vi "Set3Points.vi"(0 "Counter":i32, 5 "axis id":string[](array[string]), 7 "System number":i32, 9 "stop":bool, 11 "Z Axis Step  Size":dbl, 12 "Error In":errorcluster) -> (3 "Relative Position":dbl[](array[numeric]), 6 "3Points2DArray":dbl[][](array[numeric]), 15 "Error Out":errorcluster)   [LabVIEW 2019]
uses:
  <vilib>/Analysis/Matrix/Datatypes/RealMatrix.ctl
  <vilib>/Analysis/Matrix/Numeric/Conversions/Matrix To Array - RM.vi
  <vilib>/Analysis/Matrix/NI_Matrix.lvlib
panel:
  in  "3Points":T1
  in  "zRandom":T1
  out "Iteration":i32
  out "MaxRandomNum":dbl
  out "zrandArray":dbl[][](array[numeric])
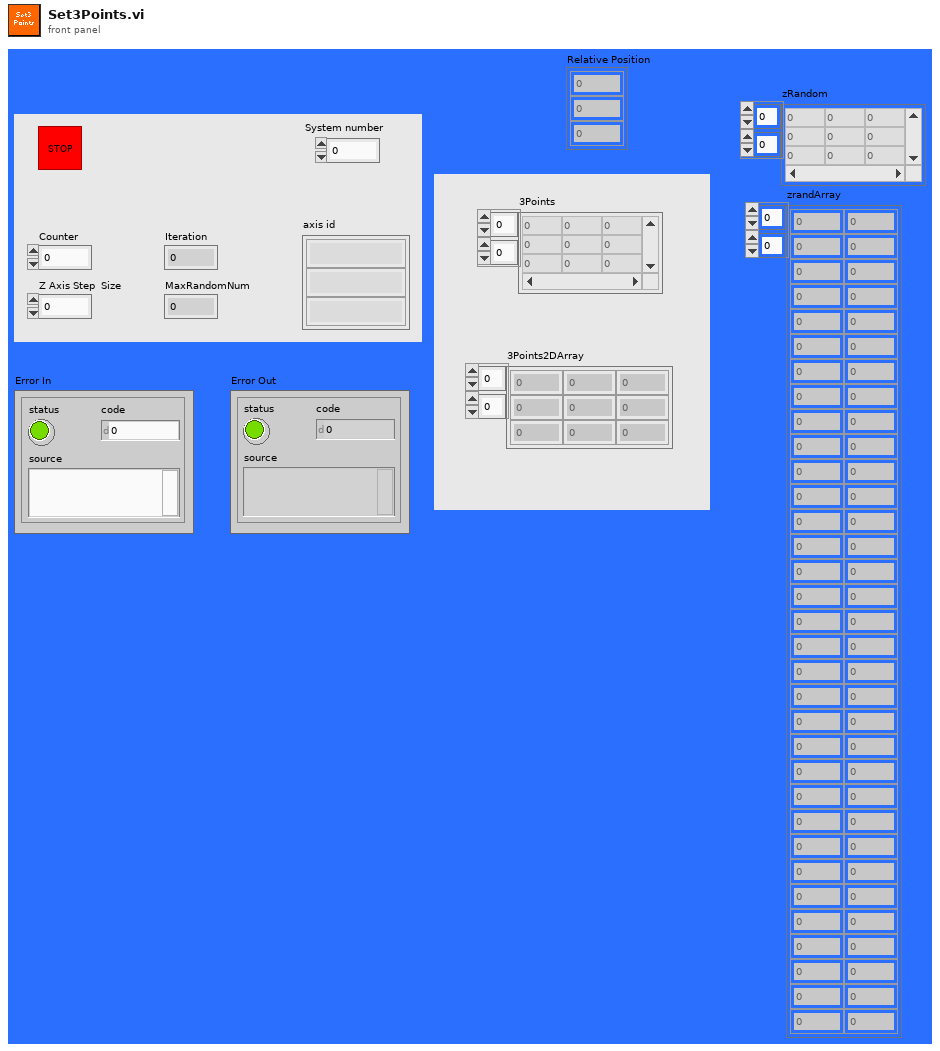
[diagram p1: front panel]
types:
  T1 = typedef "NI_Matrix.lvlib/RealMatrix.ctl" = dbl[][]
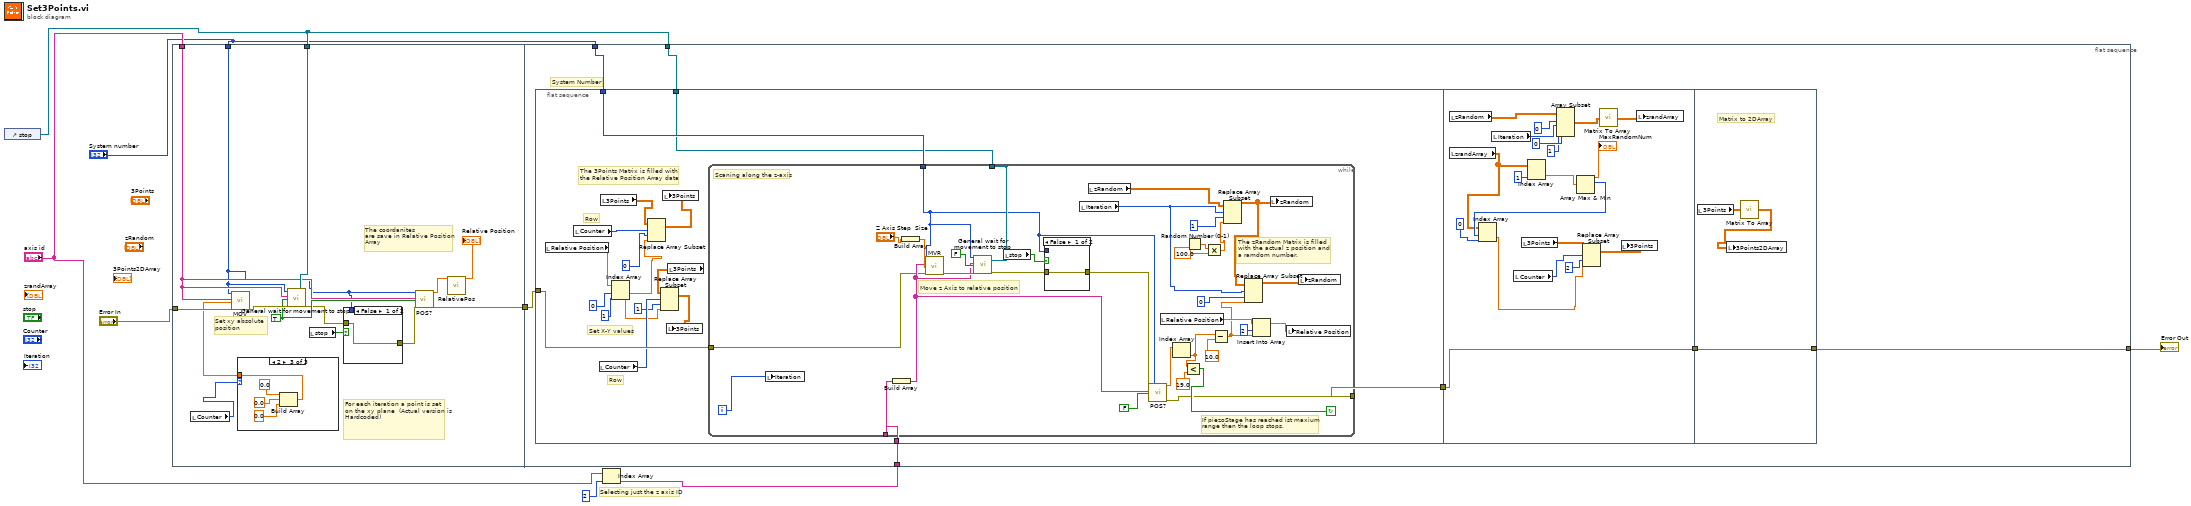
[diagram p0: block diagram]
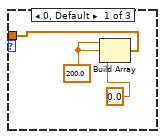
[diagram p2: hidden frame]
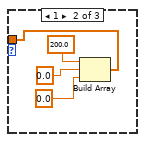
[diagram p3: hidden frame]
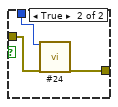
[diagram p4: hidden frame]
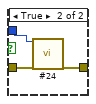
[diagram p5: hidden frame]
diagram:
  # "Selecting just the z axis ID"
  n1 = control-ref of="stop"() -> (w2:refnum<vi>)
  n2 = flat-sequence {
    tunnel: "Error In" -> [w22]
    tunnel: w2 -> [w20]
    tunnel: "axis id" -> [w18]
    tunnel: "System number" -> [w12]
    tunnel: [w19] -> w8
    tunnel: w8 -> [w44]
    tunnel: "System number" -> [w43]
    tunnel: w2 -> [w42]
    tunnel: w4 -> [w41]
    tunnel: [w39] -> w3
    frame #0 {
      w17 = TRUE ("All axes?")
      # "The coordanites\nare save in Relative Position \nArray"
      # "For each iteration a point is set\non the xy plane  (Actual version is Hardcoded)"
      # "Set xy absolute\nposition"
      n3 = local read "Counter"() -> (w9:i32)
      n4 = case shown="2" w9 {
        tunnel: [w23 w26 w30] -> w10
        frame 0, Default {
          w25 = 200.0 ("element")
          n5 = Build Array(w25, w25, 0.0 ("element")) -> (w23:dbl[])
        }
        frame 1 {
          n6 = Build Array(200.0, 0.0, 0.0) -> (w26:dbl[])
        }
        frame 2 {
          n7 = Build Array(0.0, 0.0, 0.0) -> (w30:dbl[])
        }
      }
      n8 = call "MOV.vi"("System no."=w12, "Axes to move"=w18, "Position values"=w10, "error in"=w22) -> ("error out"=w21:errorcluster)  [unwired: 15 in]
      n9 = call "General wait for movement to stop.vi"("System no."=w12, "Axes to wait for"=w18, "All axes?"=w17, "error in"=w21, "Stop refnum"=w20) -> ("error out"=w13:errorcluster)  [unwired: 13 in, 1 out]
      n10 = local read "stop"() -> (w14:bool)
      n11 = case shown="False" w14 {
        tunnel: w13 -> [w34 w37]
        tunnel: w12 -> [_ w36]
        tunnel: [w34 w35] -> w11
        frame False {
        }
        frame True {
          n12 = call "#24.vi"("System no."=w36, "error in"=w37) -> ("error out"=w35:errorcluster)  [unwired: 17 in]
        }
      }
      n13 = call "POS?.vi"("System no."=w12, "Axes to query"=w18, "All axes?"=w17, "error in"=w11) -> ("Position"=w16:dbl[], "error out"=w19:errorcluster)  [unwired: 14 in]
      n14 = call "RelativePos.vi"("AxisPos"=w16) -> ("Relative Position"=→"Relative Position":dbl[])  [unwired: 10 in]
    }
    frame #1 {
      # "System Number"
      n15 = flat-sequence {
        tunnel: w44 -> [w62]
        tunnel: w43 -> [w61]
        tunnel: w42 -> [w60]
        tunnel: w41 -> [w56]
        tunnel: [w55] -> w40
        tunnel: w40 -> [w113]
        tunnel: [w113] -> w38
        tunnel: [w121] -> w39
        tunnel: w38 -> [w121]
        frame #0 {
          # "The 3Points Matrix is filled with \nthe Relative Position Array data"
          # "Row"
          # "Row"
          # "Set X-Y values"
          n16 = local read "Relative Position"() -> (w59:dbl[])
          n17 = local read "Counter"() -> (w48:i32)
          n18 = local read "Counter"() -> (w53:i32)
          n19 = local read "3Points"() -> (w49:T1)
          n20 = Index Array(array=w59, index #1=0 ("index"), index #2=1 ("index")) -> (element #1=w46:dbl, element #2=w51:dbl)
          n21 = Replace Array Subset(array=w49, new element=w46, index (row)=w48, index (col)=0 ("index (row)")) -> (w45:T1)
          n22 = local write "3Points"(w45) -> ()
          n23 = local read "3Points"() -> (w54:T1)
          n24 = Replace Array Subset(array=w54, new element=w51, index (row)=w53, index (col)=1 ("disabled index (col)")) -> (w50:T1)
          n25 = local write "3Points"(w50) -> ()
          n26 = while {
            tunnel: w56 -> [w95]
            tunnel: w62 -> [w81]
            tunnel: w61 -> [w86]
            tunnel: [w91] -> _
            tunnel: w60 -> [w91]
            tunnel: [w79] -> w55
            i -> [w73]
            stop <- w82 continue-if-true
            # "The zRandom Matrix is filled\nwith the actual z position and \na ramdom number."
            # "If piezoStage has reached ist maxium \nrange then the loop stops."
            # "Scaning along the z-axis"
            # "Move z Axis to relative position"
            n27 = local write "Iteration"(w73) -> ()
            n28 = Build Array(w95) -> (w85:string[])
            n29 = Build Array("Z Axis Step  Size") -> (w93:dbl[])
            n30 = call "MVR.vi"("System no."=w86, "Axes to move"=w85, "Position values"=w93, "error in"=w81) -> ("error out"=w92:errorcluster)  [unwired: 15 in]
            n31 = call "General wait for movement to stop.vi"("System no."=w86, "Axes to wait for"=w85, "All axes?"=FALSE, "error in"=w92, "Stop refnum"=w91) -> ("error out"=w89:errorcluster)  [unwired: 13 in, 1 out]
            n32 = local read "stop"() -> (w88:bool)
            n33 = case shown="False" w88 {
              tunnel: w89 -> [w96 w99]
              tunnel: w86 -> [_ w98]
              tunnel: [w96 w97] -> w87
              frame False {
              }
              frame True {
                n34 = call "#24.vi"("System no."=w98, "error in"=w99) -> ("error out"=w97:errorcluster)  [unwired: 17 in]
              }
            }
            n35 = local read "Iteration"() -> (w75:i32)
            n36 = local read "zRandom"() -> (w78:T1)
            n37 = call "POS?.vi"("System no."=w86, "Axes to query"=w85, "All axes?"=FALSE, "error in"=w87) -> ("Position"=w69:dbl[], "error out"=w79:errorcluster)  [unwired: 14 in]
            n38 = local read "Relative Position"() -> (w70:dbl[])
            n39 = Index Array(array=w69) -> (element=w68:dbl)  [unwired: 1 in]
            n40 = Less?(x=w68, y=19.0) -> (x < y?=w82:bool)
            n41 = Random Number (0-1)() -> (number: 0 to 1=w66:dbl)
            n42 = Multiply(x=w66, y=100.0) -> (x*y=w64:dbl)
            n43 = Subtract(x=w68, y=10.0) -> (x-y=w67:dbl)
            n44 = Replace Array Subset(array=w78, new element=w64, index (row)=w75, index (col)=1 ("disabled index (col)")) -> (w63:T1)
            n45 = Replace Array Subset(array=w63, new element=w67, index (row)=w75, index (col)=0 ("disabled index (col)")) -> (w76:T1)
            n46 = Insert Into Array(array=w70, index=2, new element=w67) -> (w72:dbl[])
            n47 = local write "zRandom"(w63) -> ()
            n48 = local write "Relative Position"(w72) -> ()
            n49 = local write "zRandom"(w76) -> ()
          }
        }
        frame #1 {
          n50 = local read "zRandom"() -> (w106:T1)
          n51 = local read "zrandArray"() -> (w114:dbl[][])
          n52 = local read "Iteration"() -> (w104:i32)
          n53 = local read "Counter"() -> (w110:i32)
          n54 = local read "3Points"() -> (w111:T1)
          n55 = Index Array(array=w114, index (col)=1 ("disabled index (col)")) -> (element=w109:dbl[])  [unwired: 1 in]
          n56 = Array Subset(array=w106, index (row)=0 ("row 1"), length (row)=w104, index (col)=0 ("column N"), length (col)=1 ("column N")) -> (w103:T1)
          n57 = Array Max & Min(array=w109) -> (max value=→"MaxRandomNum":dbl, max index (indices)=w116:i32)  [unwired: 2 out]
          n58 = Index Array(array=w114, index (row)=w116, index (col)=0 ("disabled index (col)")) -> (element=w107:dbl)
          n59 = Replace Array Subset(array=w111, new element=w107, index (row)=w110, index (col)=2 ("disabled index (col)")) -> (w112:T1)
          n60 = call-poly <vilib>:"Matrix To Array.vi"("Real Matrix"=w103) -> ("Real 2D Array"=w102:dbl[][])
          n61 = local write "3Points"(w112) -> ()
          n62 = local write "zrandArray"(w102) -> ()
        }
        frame #2 {
          # "Matrix to 2DArray"
          n63 = local read "3Points"() -> (w120:T1)
          n64 = call-poly <vilib>:"Matrix To Array.vi"("Real Matrix"=w120) -> ("Real 2D Array"=w119:dbl[][])
          n65 = local write "3Points2DArray"(w119) -> ()
        }
      }
    }
  }
  n66 = Index Array(array="axis id", index=2) -> (element=w4:string)
  "Error Out" <- w3
